vi "Get Addresses for Deactivation.vi"(8 "error in (no error)":errorcluster, 10 "config file refnum in":T1, 11 "IED in":refnum<class "IED.lvclass">) -> (0 "error out":errorcluster, 2 "config file refnum out":T1, 3 "IED out":refnum<class "IED.lvclass">)   [LabVIEW 2015, in "IED Actor.lvlib" / "IED.lvclass"]
uses:
  IED.lvclass
  <vilib>/Utility/config.llb/Config Data RefNum.ctl
  IED.lvclass/IED.ctl
  <vilib>/Utility/config.llb/Read Key (U32).vi
  <vilib>/Modbus/master/Modbus Master.lvclass
  <vilib>/Utility/config.llb/NI_LVConfig.lvlib
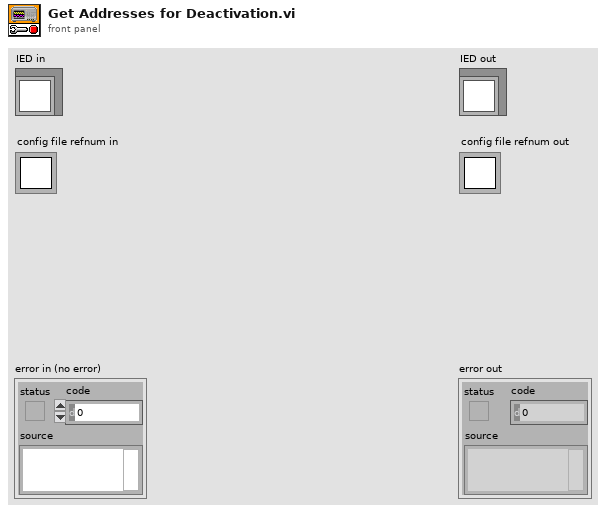
[diagram p1: front panel]
types:
  T1 = typedef "NI_LVConfig.lvlib/Config Data RefNum.ctl" = refnum<k1>
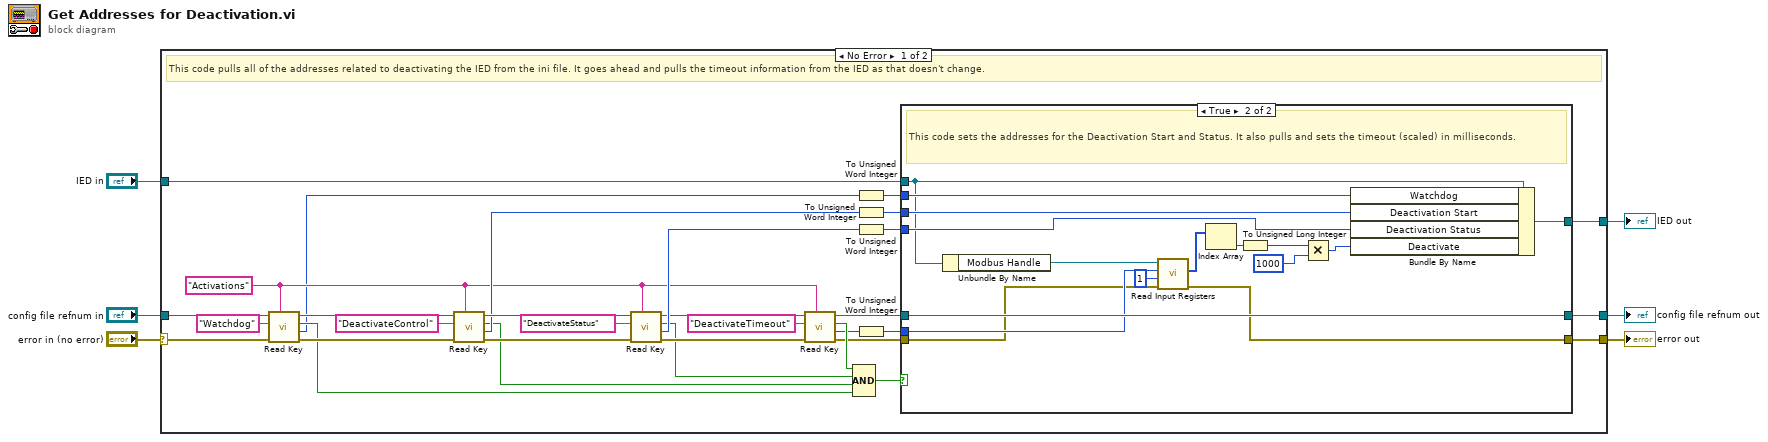
[diagram p0: block diagram]
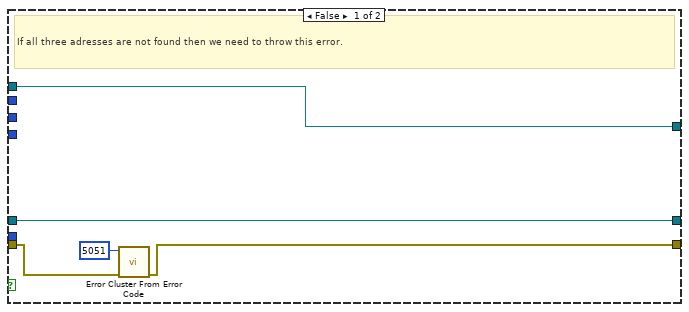
[diagram p2: hidden frame]
diagram:
  n1 = case shown="No Error" "error in (no error)" {
    selector: "error in (no error)" -> [w14 w62]
    tunnel: [w21 w62] -> w3
    tunnel: [w20 w61] -> w4
    tunnel: "IED in" -> [w22 w61]
    tunnel: "config file refnum in" -> [w13 w60]
    tunnel: [w19 w60] -> w1
    frame No Error {
      w12 = "Activations" ("section")
      # "This code pulls all of the addresses related to deactivating the IED from the ini file. It goes ahead and pulls the timeout information from the IED as that doesn't change."
      n2 = call-poly <vilib>:"Read Key.vi"("section"=w12, "error in (no error)"=w14, "key"="Watchdog", "refnum"=w13) -> ("error out"=w15:errorcluster, "value"=w8:u32, "found?"=w10:bool, "refnum out"=w16:T1)  [unwired: 4 in]
      n3 = call-poly <vilib>:"Read Key.vi"("section"=w12, "error in (no error)"=w15, "key"="DeactivateControl", "refnum"=w16) -> ("error out"=w37:errorcluster, "value"=w34:u32, "found?"=w27:bool, "refnum out"=w36:T1)  [unwired: 4 in]
      n4 = call-poly <vilib>:"Read Key.vi"("section"=w12, "error in (no error)"=w37, "key"="DeactivateStatus", "refnum"=w36) -> ("error out"=w31:errorcluster, "value"=w33:u32, "found?"=w28:bool, "refnum out"=w32:T1)  [unwired: 4 in]
      n5 = call-poly <vilib>:"Read Key.vi"("section"=w12, "error in (no error)"=w31, "key"="DeactivateTimeout", "refnum"=w32) -> ("error out"=w24:errorcluster, "value"=w17:u32, "found?"=w29:bool, "refnum out"=w25:T1)  [unwired: 4 in]
      n6 = Compound Arithmetic op=AND(w29, w28, w27, w10) -> (w26:bool)
      n7 = To Unsigned Word Integer(number=w8) -> (unsigned 16bit integer=w7:u16)
      n8 = To Unsigned Word Integer(number=w34) -> (unsigned 16bit integer=w9:u16)
      n9 = To Unsigned Word Integer(number=w33) -> (unsigned 16bit integer=w23:u16)
      n10 = To Unsigned Word Integer(number=w17) -> (unsigned 16bit integer=w18:u16)
      n11 = case shown="True" w26 {
        tunnel: w25 -> [w39 w55]
        tunnel: w24 -> [w43 w46]
        tunnel: w18 -> [_ w54]
        tunnel: w9 -> [_ w59]
        tunnel: w23 -> [_ w58]
        tunnel: w22 -> [w40 w49]
        tunnel: [w41 w44] -> w21
        tunnel: [w40 w57] -> w20
        tunnel: [w39 w55] -> w19
        tunnel: w7 -> [_ w56]
        frame False {
          # "If all three adresses are not found then we need to throw this error."
          n12 = call <vilib>:"Error Cluster From Error Code.vi"("error in (no error)"=w43, "error code (0)"=5051) -> ("error out"=w41:errorcluster)  [unwired: 7 in]
        }
        frame True {
          # "This code sets the addresses for the Deactivation Start and Status. It also pulls and sets the timeout (scaled) in milliseconds."
          n13 = Unbundle By Name(w49) -> ("Modbus Handle"=w45:refnum<class "Modbus Master.lvclass">)
          n14 = call-dynamic "Read Input Registers.vi"("error in (no error)"=w46, "number of input registers"=u16 1, "starting address"=w54, "Modbus master in"=w45) -> ("error out"=w44:errorcluster, "register values"=w52:u16[])  [unwired: 5 in, 1 out]
          n15 = Index Array(array=w52) -> (element=w53:u16)  [unwired: 1 in]
          n16 = To Unsigned Long Integer(number=w53) -> (unsigned 32bit integer=w50:u32)
          n17 = Multiply(x=w50, y=u32 1000) -> (x*y=w48:u32)
          n18 = Bundle By Name(cluster=w49, "Watchdog"=w56, "Deactivation Start"=w59, "Deactivation Status"=w58, "Deactivate"=w48) -> (w57:refnum<class "IED.lvclass">)
        }
      }
    }
    frame Error {
    }
  }
  "error out" <- w3
  "IED out" <- w4
  "config file refnum out" <- w1
